vi "AssembleBLMultiplotScript.vi"() -> ()   [LabVIEW 2013]
uses:
  minAndMax.ctl
  AutoManualNumber.ctl
  margins.ctl
  axisName.ctl
  ticsAndGrids.ctl
  tics.ctl
  grids.ctl
panel:
  in  "lambdaBounds":T1={"Min"={"Auto"=FALSE, "Value"=0.0}, "Max"={"Auto"=FALSE, "Value"=0.6}}
  in  "U/UrefBounds":T1={"Min"={"Auto"=FALSE, "Value"=0.0}, "Max"={"Auto"=FALSE, "Value"=1.2}}
  out "String out":string
  in  "Mapping":enum16{"Lin", "Log"}(ring)=enum."Log"
  in  "HeightAxisBounds":T1={"Min"={"Auto"=FALSE, "Value"=5.0}, "Max"={"Auto"=FALSE, "Value"=2000.0}}
  in  "jitterFraction":dbl=0.03
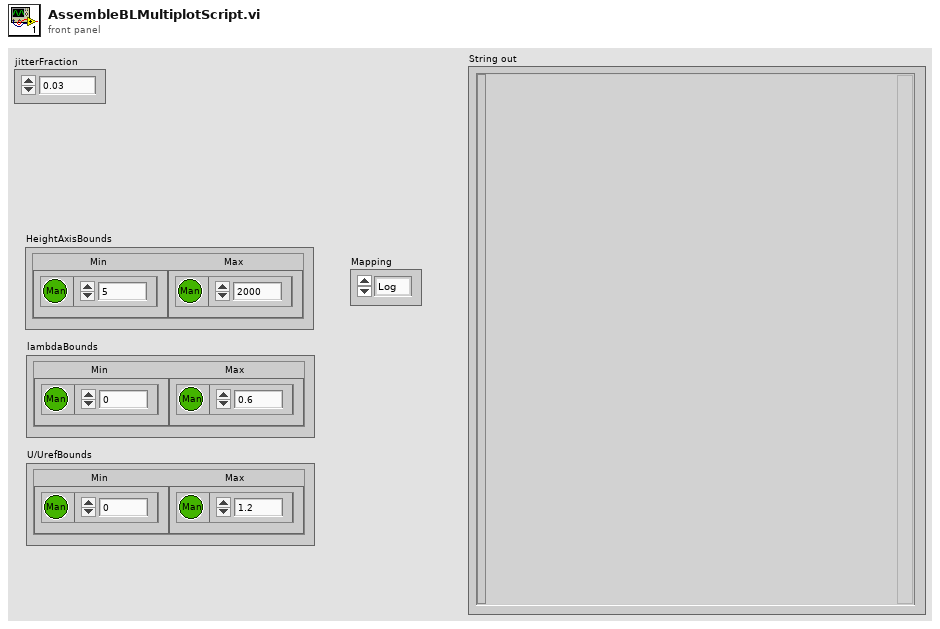
[diagram p1: front panel]
types:
  T1 = typedef "minAndMax.ctl" = cluster{"Min":T2, "Max":T2}
  T2 = typedef "AutoManualNumber.ctl" = cluster{"Auto":bool, "Value":dbl}
  T3 = typedef "axisName.ctl" = string
  T4 = typedef "ticsAndGrids.ctl" = cluster{"tics":T5, "Grids":T6, "Mapping":enum16{"Lin", "Log"}}
  T5 = typedef "tics.ctl" = cluster{"ticMin":dbl, "ticStep":dbl, "ticMax":dbl, "minorDivsPerMajor":i32, "ticSpacing":enum16{"Auto Tics", "Fixed spacing", "Fixed Minimum and Spacing", "Start, Spacing and Maximum", "Approx n Tics (rounded)"}, "ticPosition":enum16{"Inside, no mirror", "Inside, mirrored", "Outside, no mirror", "Outside, mirrored", "Invisible"}}
  T6 = typedef "grids.ctl" = cluster{"Gridlines":enum16{"No grids", "Major grid", "Minor grid", "Major and Minor"}, "Zeroaxis":enum16{"No zero axis", "Show zero axis"}}
  T7 = typedef "margins.ctl" = cluster{"Top":dbl, "Bottom":dbl, "Left":dbl, "Right":dbl}
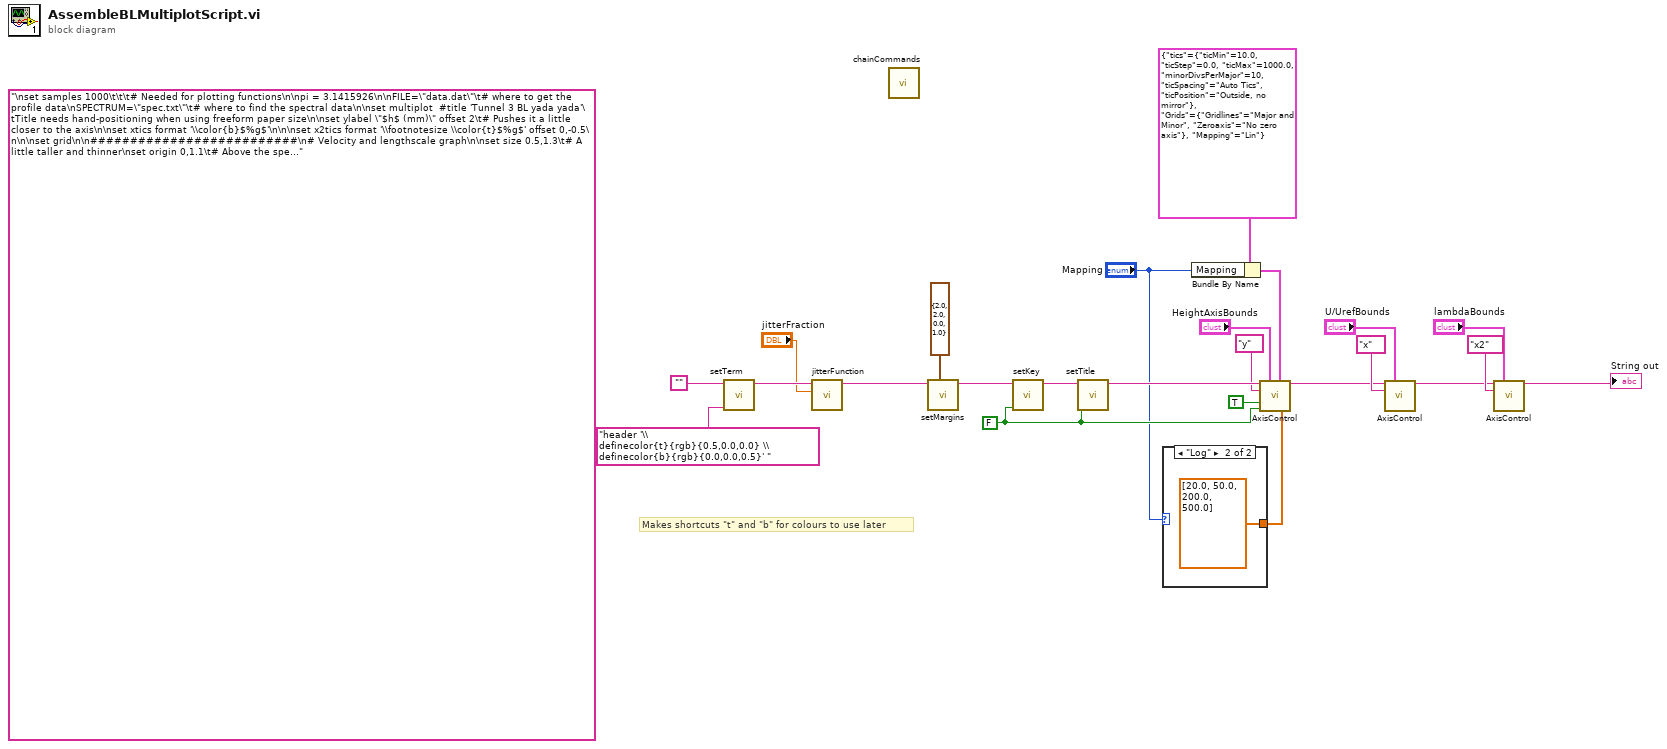
[diagram p0: block diagram]
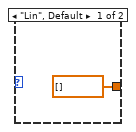
[diagram p2: hidden frame]
diagram:
  w10 = FALSE ("Set?")
  (unwired) "\nset samples 1000\t\t\t# Needed for plotting functions\n\npi = 3.1415926\n\nFILE=\"data.dat\"\t# where to get the profile data\nSPECTRUM=\"spec.txt\"\t# where to find the spectral data\n\nset multiplot  #title 'Tunnel 3 BL yada yada'\tTitle needs hand-positioning when using freeform paper size\n\nset ylabel \"$h$ (mm)\" offset 2\t# Pushes it a little closer to the axis\n\nset xtics format '\\color{b}$%g$'\n\n\nset x2tics format '\\footnotesize \\color{t}$%g$' offset 0,-0.5\n\n\nset grid\n\n##########################\n# Velocity and lengthscale graph\n\nset size 0.5,1.3\t# A little taller and thinner\nset origin 0,1.1\t# Above the spectrum\n\nset xlabel '\\color{b}{$U/U_{ref}$}'\nset xrange [0:1.2]\nset xtics  0,0.2,1.0\n\nset x2label '\\footnotesize \\color{t}{$\\lambda(U)$ (m)}' offset 0,-0.5\nset x2range [0:0.6]\nset x2tics  0,0.1,0.5\n\n\nplot FILE index 0 using 1:(jittered($2)) axes x1y1 title 'Velocity' w points lc rgb \"#000080\" pt 6 ps 1.5, \\\nFILE index 3 using 1:(jittered($2)) axes x2y1 title 'Lengthscale' w points lc rgb \"#800000\" pt 2 ps 0.8\n\n##########################\n# TI and sigma graph\n\nset size 0.5,1.3\t\t\t# A little taller and thinner\nset origin 0.5,1.1\t\t\t# In the bottom-left corner\n\nset format y \"\"\nunset ylabel\n\nset xlabel '\\color{b}{$Turbulence~Intensity$~(\\%)}'\nset xrange [0:30]\nset xtics 0,5,30\n\nset x2label '\\footnotesize \\color{t}{$\\sigma(U)/U_{ref}$}' offset 0,-0.5\nset x2range [0:0.12]\nset x2tics 0,0.02,0.1\n\nplot FILE index 1 using 1:(jittered($2)) axes x1y1 title 'Turbulence' w points lc rgb '#000080' pt 6 ps 1.5, \\\nFILE index 2 using 1:(jittered($2)) axes x2y1 title 'sigma/U' w points lc rgb '#800000' pt 2 ps 0.8\n\n\n##########################\n# And now the Spectrum and (gnuplot-calculated, for now, fit)\nset size 1,1\nset origin 0,0\n\nset title 'Longitudinal velocity power spectrum' offset 0, -0.5\nset xlabel '$f$ (Hz)'\nset ylabel '$f.S(f)$'\n\nunset x2label\nunset x2tics\n\nset logscale x\nset logscale y\n\nset xrange [*:*]\nset yrange [*:*]\n\nset xtics autofreq nomirror\n\nset ytics autofreq nomirror\nset format y \"\"\nset ytics scale 1\nset mxtics \nset mytics\n\n\nsigsq=0.54\nlu=1\nU= 10\n\n# Fit equation from VELSPEC document:\nfvonK(x)=sigsq*4*(x*lu/U)/(1+((2*pi*1.339)**2)*(x*lu/U)**2)**(5./6)\t# 1.339 is a constant (fudge factor?), from vK himself\n\n# Can limit the range of the fit with a [fmin:fmax] type command...\n# sigsq should not really be a DOF; but it's interesting (and heartening) to see it come out the same as from the time series\nfit fvonK(x) \"spec.txt\" u 1:($1*$2) via lu\n\n\nset key inside bottom left spacing 1.2\n\n# form f.S(f) using maths as you plot. Could save f.S(f) from Measurement instead...\nplot SPECTRUM using 1:($1*$2) title 'Tunnel data, h=XXmm' axes x1y1 w  points lc rgb '#A50021' pt 7 ps 1, \\\nfvonK(x) title 'vK fit' w lines ls 1 lc rgb \"#000099\"\n\nunset multiplot\t# All done :-)\n"
  # "Makes shortcuts \"t\" and \"b\" for colours to use later"
  n1 = call "setTerm.vi"("Additional Terminal Options"="header '\\definecolor{t}{rgb}{0.5,0.0,0.0} \\definecolor{b}{rgb}{0.0,0.0,0.5}' ", "String in"="") -> ("String out"=w22:string)  [unwired: 8 in, 1 out]
  n2 = call "jitterFunction.vi"("jitterFraction"="jitterFraction", "String in"=w22) -> ("String out"=w20:string)  [unwired: 8 in, 1 out]
  n3 = call "chainCommands.vi"() -> ()  [unwired: 11 in, 1 out]
  n4 = call "setMargins.vi"("Margins"=T7 {"Top"=2.0, "Bottom"=2.0, "Left"=0.0, "Right"=1.0}, "String in"=w20) -> ("String out"=w18:string)  [unwired: 8 in, 1 out]
  n5 = call "setKey.vi"("Set?"=w10, "String in"=w18) -> ("String out"=w17:string)  [unwired: 8 in, 1 out]
  n6 = call "setTitle.vi"("Set?"=w10, "String in"=w17) -> ("String out"=w16:string)  [unwired: 8 in, 1 out]
  n7 = case shown="\"Log\"" "Mapping" {
    tunnel: [dbl[] [] ("AdditionalTics") dbl[] [20.0, 50.0, 200.0, 500.0] ("AdditionalTics")] -> w9
    frame "Lin", Default {
    }
    frame "Log" {
    }
  }
  n8 = Bundle By Name(cluster=T4 {"tics"={"ticMin"=10.0, "ticStep"=0.0, "ticMax"=1000.0, "minorDivsPerMajor"=10, "ticSpacing"=enum."Auto Tics", "ticPosition"=enum."Outside, no mirror"}, "Grids"={"Gridlines"=enum."Major and Minor", "Zeroaxis"=enum."No zero axis"}, "Mapping"=enum."Lin"} ("ticsAndGrids"), "Mapping"="Mapping") -> (w12:T4)
  n9 = call "AxisControl.vi"("String in"=w16, "AxisBounds"="HeightAxisBounds", "ticsAndGrids"=w12, "Axis"=T3 "y", "ShowNumbers?"=TRUE, "ShowLabel?"=w10, "AdditionalTics"=w9) -> ("String out"=w5:string)  [unwired: 7 in, 1 out]
  n10 = call "AxisControl.vi"("String in"=w5, "AxisBounds"="U/UrefBounds", "Axis"=T3 "x") -> ("String out"=w4:string)  [unwired: 11 in, 1 out]
  n11 = call "AxisControl.vi"("String in"=w4, "AxisBounds"="lambdaBounds", "Axis"=T3 "x2") -> ("String out"=→"String out":string)  [unwired: 11 in, 1 out]
